vi "update map.vi"(0 "coordinates":i8[][](array[numeric]), 2 "Array in":refnum<vi>) -> ()   [LabVIEW 2020]
doc: "update the map by only turn on the button at coordinate element of the input array(n rows 2 columns)"
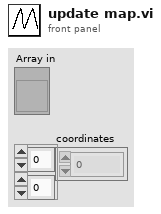
[diagram p1: front panel]
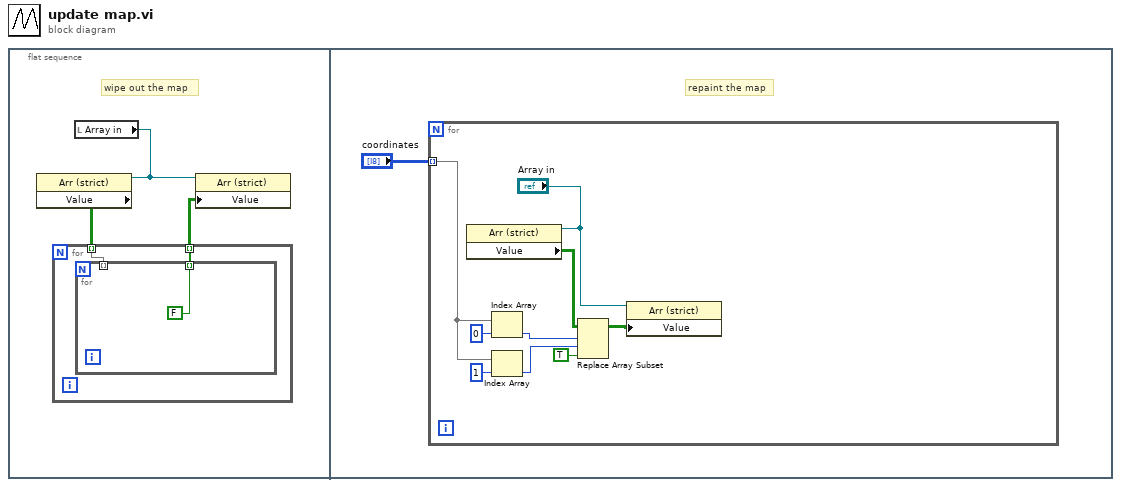
[diagram p0: block diagram]
diagram:
  n1 = flat-sequence {
    frame #0 {
      # "wipe out the map"
      n2 = local read "Array in"() -> (w3:refnum<vi>)
      n3 = property class="Arr (strict)"(reference=w3) -> ("Value"=w2:bool[][])  [unwired: 1 in, 2 out]
      n4 = for {
        tunnel: w2 -> [w5] mode=indexing
        tunnel: [w4] -> w1 mode=indexing
        n5 = for {
          tunnel: w5 -> [_] mode=indexing
          tunnel: [FALSE] -> w4 mode=indexing
        }
      }
      n6 = property class="Arr (strict)"(reference=w3, "Value"=w1) -> ()  [unwired: 1 in, 2 out]
    }
    frame #1 {
      # "repaint the map"
      n7 = for {
        tunnel: "coordinates" -> [w14] mode=indexing
        n8 = property class="Arr (strict)"(reference="Array in") -> ("Value"=w8:bool[][])  [unwired: 1 in, 2 out]
        n9 = Index Array(array=w14, index=0) -> (element=w13:i8)
        n10 = Index Array(array=w14, index=1) -> (element=w12:i8)
        n11 = Replace Array Subset(array=w8, new element=TRUE ("new element/subarray"), index (row)=w13, index (col)=w12) -> (w10:bool[][])
        n12 = property class="Arr (strict)"(reference="Array in", "Value"=w10) -> ()  [unwired: 1 in, 2 out]
      }
    }
  }
